vi "szablon odometry_filtered_local.vi"() -> ()   [LabVIEW 2015, in "Biblioteka moduł map v3.lvlib" / "Zmienne.lvlib"]
uses:
  Zmienne.lvlib
  szablon odometry_filtered_local.ctl
panel:
  in  "szablon odometry/filtered/local":T1
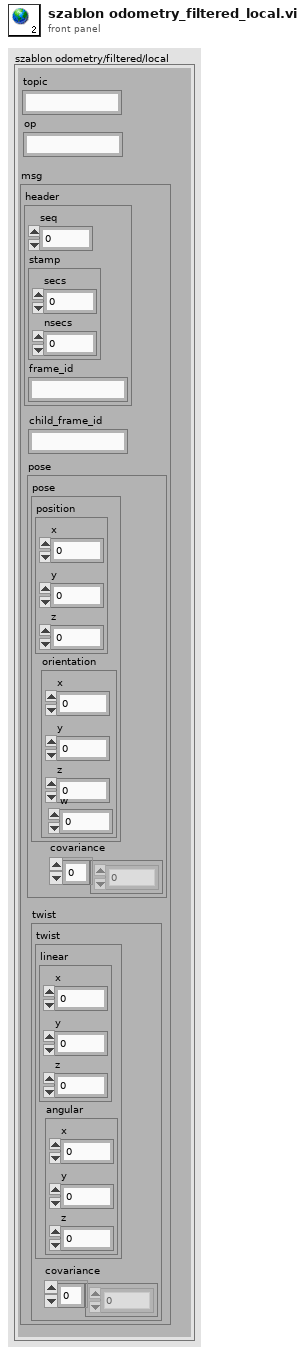
[diagram p1: front panel]
types:
  T1 = typedef "Biblioteka moduł map v3.lvlib/Zmienne.lvlib/szablon odometry_filtered_local.ctl" = cluster{"topic":string, "msg":cluster{"header":cluster{"seq":u32, "stamp":cluster{"secs":u32, "nsecs":i32}, "frame_id":string}, "child_frame_id":string, "pose":cluster{"pose":cluster{"position":cluster{"y":dbl, "z":dbl, "x":dbl}, "orientation":cluster{"y":dbl, "z":dbl, "x":dbl, "w":dbl}}, "covariance":dbl[]}, "twist":cluster{"twist":cluster{"linear":cluster{"y":dbl, "z":dbl, "x":dbl}, "angular":cluster{"y":dbl, "z":dbl, "x":dbl}}, "covariance":dbl[]}}, "op":string}
diagram:
